vi "Accumulate Wing Sector Pixel Values (FPGA).vi"(1 "Right Wing Sector Pixel Count":u16[](array[numeric]), 5 "NumWingSectors":u8, 6 "Right Wing Sector Pixel Values":u16[](array[numeric]), 7 "Left Wing Sector Pixel Values":u16[](array[numeric]), 8 "Left Wing Sector Pixel Count":u16[](array[numeric]), 9 "Wing ROIs":T2, 10 "Pixel":T1) -> (0 "Right Wing Sector Pixel Values 2":u16[](array[numeric]), 2 "Left Wing Sector Pixel Values 2":u16[](array[numeric]), 3 "Left Wing Sector Pixel Count 2":u16[](array[numeric]), 4 "Right Wing Sector Pixel Count 2":u16[](array[numeric]))   [LabVIEW 2013]
uses:
  <vilib>/rvi/FXPMathLib/FxpAdd/XNode/nifxpmath_Add.xnode
  <vilib>/rvi/FXPMathLib/sim/FxpSim.dll
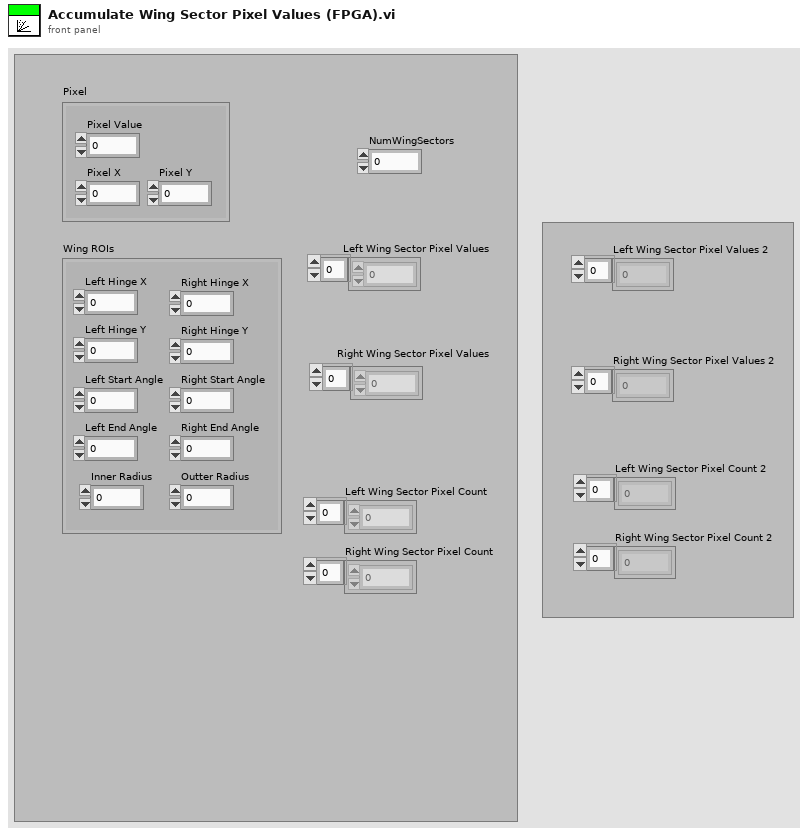
[diagram p1: front panel]
types:
  T1 = cluster{"Pixel Value":u8, "Pixel X":u16, "Pixel Y":u16}
  T2 = cluster{"Left Hinge X":u16, "Left Hinge Y":u16, "Inner Radius":u16, "Outter Radius":u16, "Right Hinge X":u16, "Right Hinge Y":u16, "Right Start Angle":i16, "Right End Angle":i16, "Left Start Angle":i16, "Left End Angle":i16}
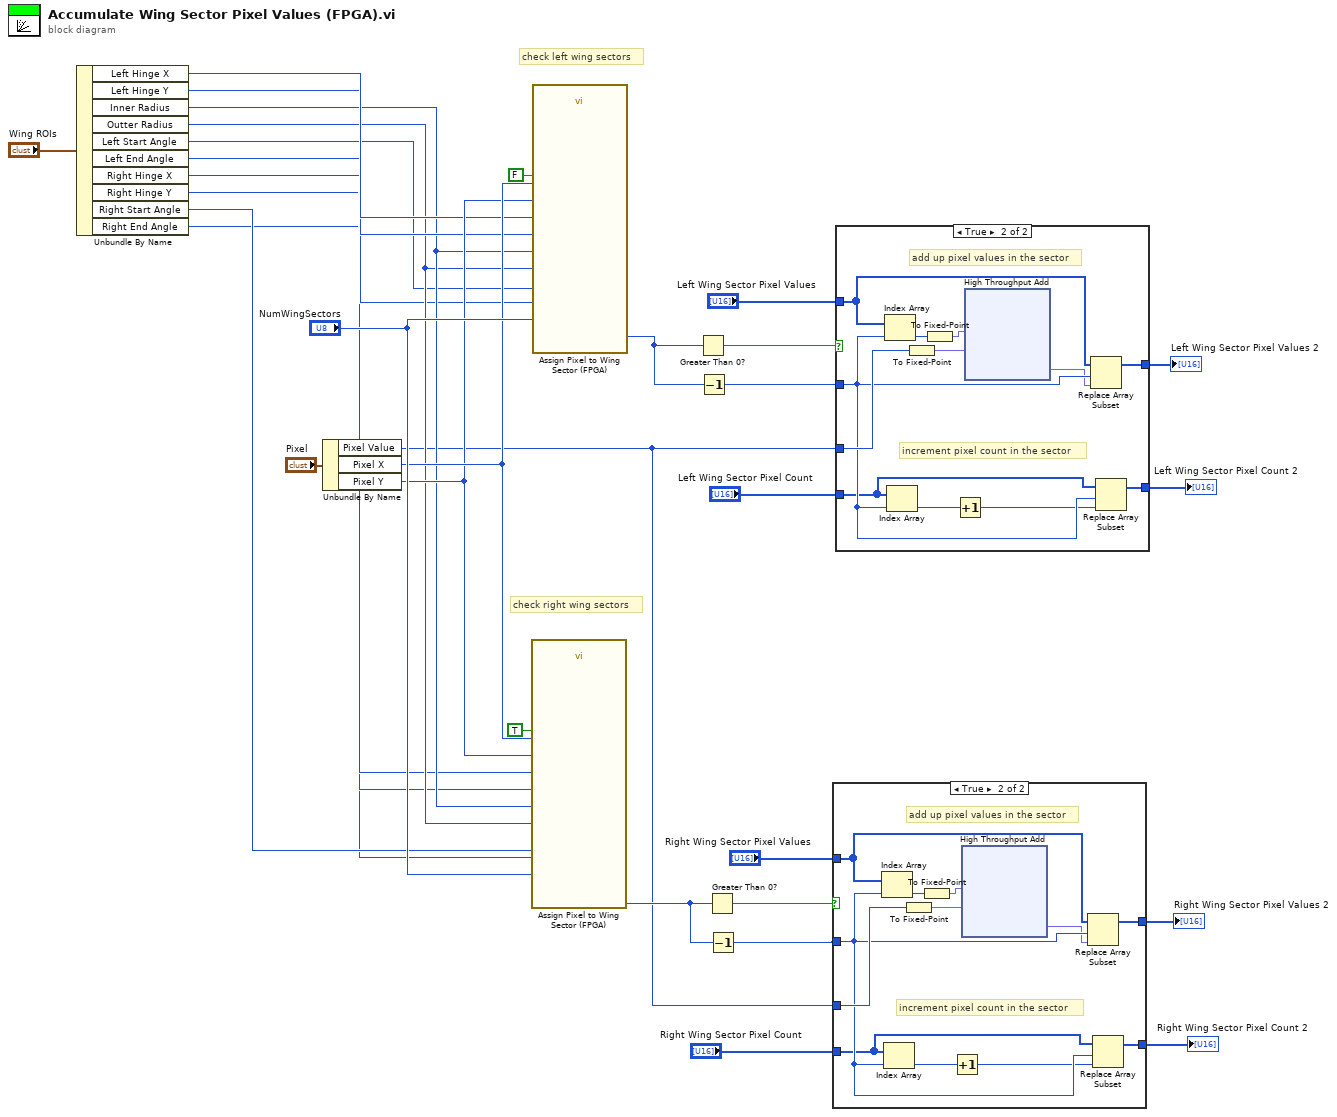
[diagram p0: block diagram]
diagram:
  # "check right wing sectors"
  # "check left wing sectors"
  n1 = Unbundle By Name("Wing ROIs") -> ("Left Hinge X"=w20:u16, "Left Hinge Y"=w19:u16, "Inner Radius"=w18:u16, "Outter Radius"=w17:u16, "Left Start Angle"=w16:i16, "Left End Angle"=w15:i16, "Right Hinge X"=w14:u16, "Right Hinge Y"=w13:u16, "Right Start Angle"=w12:i16, "Right End Angle"=w11:i16)
  n2 = Unbundle By Name("Pixel") -> ("Pixel Value"=w4:u8, "Pixel X"=w23:u16, "Pixel Y"=w22:u16)
  n3 = call "Assign Pixel to Wing Sector (FPGA).vi"(0:w11, "sector #"=TRUE ("Right Wing?"), "output valid"="NumWingSectors", 4:w17, 5:w18, "Pixel Intensity In"=w12, "Right Wing?"=w13, "Sector Parameters"=w14, "Pixel Y"=w22, "Pixel X"=w23) -> ("Pixel Intensity Out"=w26:u8)
  n4 = call "Assign Pixel to Wing Sector (FPGA).vi"(0:w15, "sector #"=FALSE ("Right Wing?"), "output valid"="NumWingSectors", 4:w17, 5:w18, "Pixel Intensity In"=w16, "Right Wing?"=w19, "Sector Parameters"=w20, "Pixel Y"=w22, "Pixel X"=w23) -> ("Pixel Intensity Out"=w28:u8)
  n5 = Greater Than 0?(x=w28) -> (x > 0?=w30:bool)
  n6 = Decrement(x=w28) -> (x-1=w27:u8)
  n7 = Greater Than 0?(x=w26) -> (x > 0?=w6:bool)
  n8 = Decrement(x=w26) -> (x-1=w5:u8)
  n9 = case shown="True" w6 {
    tunnel: "Right Wing Sector Pixel Values" -> [w34 w43]
    tunnel: w4 -> [_ w44]
    tunnel: w5 -> [_ w42]
    tunnel: [w34 w38] -> w2
    tunnel: "Right Wing Sector Pixel Count" -> [w33 w37]
    tunnel: [w33 w46] -> w1
    frame False {
      # "don't update pixel value and count in any sector\nif the pixel doesn't fall in any sector"
    }
    frame True {
      # "increment pixel count in the sector"
      # "add up pixel values in the sector"
      n10 = Index Array(array=w43, index=w42) -> (element=w45:u16)
      n11 = Index Array(array=w37, index=w42) -> (element=w36:u16)
      n12 = To Fixed-Point(number=w44) -> (fixed-point=w39:fxp<+,8,8>)  [unwired: 1 in]
      n13 = To Fixed-Point(number=w45) -> (fixed-point=w40:fxp<+,16,16>)  [unwired: 1 in]
      n14 = Increment(x=w36) -> (x+1=w35:u16)
      n15 = xnode "High Throughput Add"("x"=w40, "y"=w39) -> ("x+y"=w41:fxp<+,17,17>)
      n16 = Replace Array Subset(array=w43, new element=w41, index=w42) -> (w38:u16[])
      n17 = Replace Array Subset(array=w37, new element=w35, index=w42) -> (w46:u16[])
    }
  }
  "Right Wing Sector Pixel Values 2" <- w2
  "Right Wing Sector Pixel Count 2" <- w1
  n18 = case shown="True" w30 {
    tunnel: "Left Wing Sector Pixel Values" -> [w48 w57]
    tunnel: w4 -> [_ w58]
    tunnel: w27 -> [_ w56]
    tunnel: [w48 w52] -> w8
    tunnel: "Left Wing Sector Pixel Count" -> [w47 w51]
    tunnel: [w47 w60] -> w9
    frame False {
      # "don't update pixel value and count in any sector\nif the pixel doesn't fall in any sector"
    }
    frame True {
      # "increment pixel count in the sector"
      # "add up pixel values in the sector"
      n19 = Index Array(array=w57, index=w56) -> (element=w59:u16)
      n20 = Index Array(array=w51, index=w56) -> (element=w50:u16)
      n21 = To Fixed-Point(number=w58) -> (fixed-point=w53:fxp<+,8,8>)  [unwired: 1 in]
      n22 = To Fixed-Point(number=w59) -> (fixed-point=w54:fxp<+,16,16>)  [unwired: 1 in]
      n23 = Increment(x=w50) -> (x+1=w49:u16)
      n24 = xnode "High Throughput Add"("x"=w54, "y"=w53) -> ("x+y"=w55:fxp<+,17,17>)
      n25 = Replace Array Subset(array=w57, new element=w55, index=w56) -> (w52:u16[])
      n26 = Replace Array Subset(array=w51, new element=w49, index=w56) -> (w60:u16[])
    }
  }
  "Left Wing Sector Pixel Values 2" <- w8
  "Left Wing Sector Pixel Count 2" <- w9
